vi "Update OI Controls.vi"(7 "ControlBoth?":bool, 8 "error in (no error)":errorcluster, 9 "Disabled Controls":string[](array[string]), 10 "Enabled Controls":string[](array[string]), 11 "VI Ref":refnum<vi>) -> (0 "error out":errorcluster)   [LabVIEW 2018]
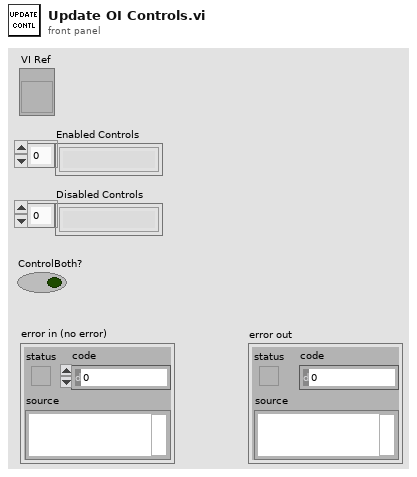
[diagram p1: front panel]
types:
  T1 = enum8{"Enabled", "Disabled", "Disabled and Grayed Out"}
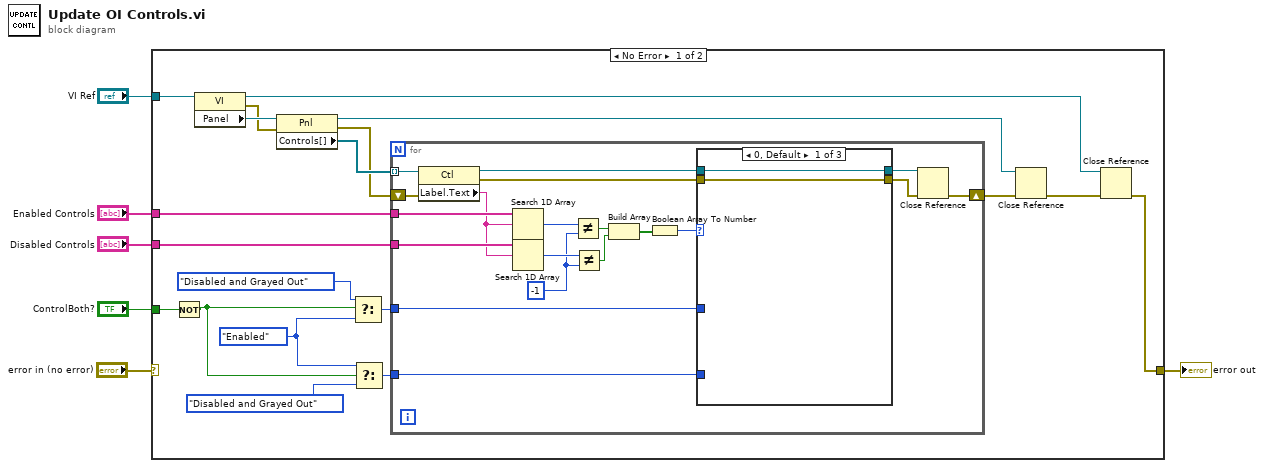
[diagram p0: block diagram]
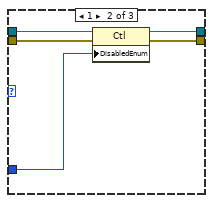
[diagram p2: hidden frame]
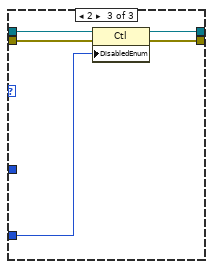
[diagram p3: hidden frame]
diagram:
  n1 = case shown="No Error" "error in (no error)" {
    selector: "error in (no error)" -> [_ w57]
    tunnel: "VI Ref" -> [w17 _]
    tunnel: "Enabled Controls" -> [w16 _]
    tunnel: "ControlBoth?" -> [w9 _]
    tunnel: "Disabled Controls" -> [w8 _]
    tunnel: [w7 w57] -> w2
    frame No Error {
      w14 = T1."Enabled" ("Disabled")
      n2 = Not(x=w9) -> (.not. x?=w12:bool)
      n3 = property class="VI"(reference=w17) -> (reference out=w18:refnum<vi>, error out=w24:errorcluster, "Panel"=w25:refnum<vi>)  [unwired: 1 in]
      n4 = property class="Pnl"(reference=w25, error in=w24) -> (reference out=w21:refnum<vi>, error out=w22:errorcluster, "Controls[]"=w23:refnum<vi>[])
      n5 = Select(t=T1."Disabled and Grayed Out" ("Disabled"), s=w12, f=w14) -> (s? t:f=w11:T1)
      n6 = Select(t=w14, s=w12, f=T1."Disabled and Grayed Out") -> (s? t:f=w10:T1)
      n7 = for {
        shift-right: [w42] -> w20
        shift-left: w22 -> [w40]
        tunnel: w23 -> [w41] mode=indexing
        tunnel: w16 -> [w37]
        tunnel: w11 -> [w31]
        tunnel: w10 -> [w30]
        tunnel: w8 -> [w36]
        w32 = -1 ("y")
        n8 = property class="Ctl"(reference=w41, error in=w40) -> (reference out=w39:refnum<vi>, error out=w38:errorcluster, "Label.Text"=w35:string)
        n9 = Search 1D Array(1D array=w37, element=w35) -> (index of element=w34:i32)  [unwired: 1 in]
        n10 = Search 1D Array(1D array=w36, element=w35) -> (index of element=w33:i32)  [unwired: 1 in]
        n11 = Not Equal?(x=w34, y=w32) -> (x != y?=w29:bool)
        n12 = Not Equal?(x=w33, y=w32) -> (x != y?=w28:bool)
        n13 = Build Array(w29, w28) -> (w27:bool[])
        n14 = Boolean Array To Number(Boolean array=w27) -> (number=w26:u32)
        n15 = case shown="0, Default" w26 {
          tunnel: [w46 w51 w56] -> w44
          tunnel: [w45 w50 w55] -> w43
          tunnel: w39 -> [w46 w49 w54]
          tunnel: w38 -> [w45 w48 w53]
          tunnel: w31 -> [_ w47 _]
          tunnel: w30 -> [_ _ w52]
          frame 0, Default {
          }
          frame 1 {
            n16 = property class="Ctl"(reference=w49, error in=w48, "DisabledEnum"=w47) -> (reference out=w51:refnum<vi>, error out=w50:errorcluster)
          }
          frame 2 {
            n17 = property class="Ctl"(reference=w54, error in=w53, "DisabledEnum"=w52) -> (reference out=w56:refnum<vi>, error out=w55:errorcluster)
          }
        }
        n18 = Close Reference(reference=w44, error in (no error)=w43) -> (error out=w42:errorcluster)
      }
      n19 = Close Reference(reference=w21, error in (no error)=w20) -> (error out=w19:errorcluster)
      n20 = Close Reference(reference=w18, error in (no error)=w19) -> (error out=w7:errorcluster)
    }
    frame Error {
    }
  }
  "error out" <- w2
